vi "Get Substrings & Calculate CRC.vi"(8 "error in (no error)":errorcluster, 11 "Data In":string) -> (0 "error out":errorcluster, 2 "Analogs":string, 3 "Switches":string)   [LabVIEW 2015]
uses:
  <vilib>/Utility/error.llb/Error Cluster From Error Code.vi
  Inline CRC/CRC SubVIs/Wrappers/CRC-8-Maxim 1-Wire (DOW).vi
  <vilib>/ErrorRing/Error Ring.xnode
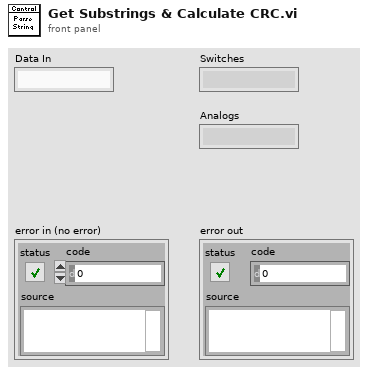
[diagram p1: front panel]
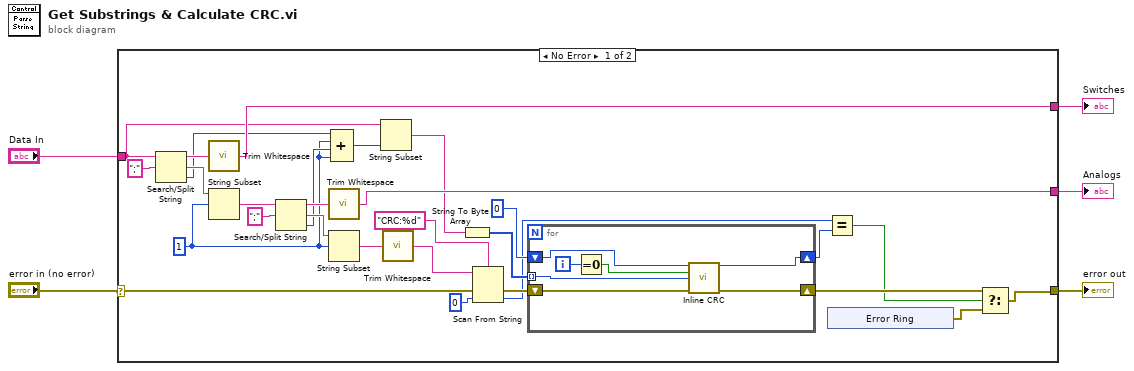
[diagram p0: block diagram]
diagram:
  n1 = case shown="No Error" "error in (no error)" {
    selector: "error in (no error)" -> [w10 w47]
    tunnel: [w32 _] -> w5
    tunnel: [w31 _] -> w4
    tunnel: "Data In" -> [w20 _]
    tunnel: [w8 w47] -> w2
    frame No Error {
      w21 = 1 ("offset (0)")
      n2 = Search/Split String(string=w20, search string/char (-)=";") -> (substring before match=w28:string, match + rest of string=w25:string, offset of match=w23:i32)  [unwired: 1 in]
      n3 = call <vilib>:"Trim Whitespace.vi"("string"=w28) -> ("trimmed string"=w31:string)  [unwired: 1 in]
      n4 = String Subset(string=w25, offset (0)=w21) -> (substring=w24:string)  [unwired: 1 in]
      n5 = Search/Split String(string=w24, search string/char (-)=";") -> (substring before match=w29:string, match + rest of string=w27:string, offset of match=w22:i32)  [unwired: 1 in]
      n6 = call <vilib>:"Trim Whitespace.vi"("string"=w29) -> ("trimmed string"=w32:string)  [unwired: 1 in]
      n7 = String Subset(string=w27, offset (0)=w21) -> (substring=w26:string)  [unwired: 1 in]
      n8 = Compound Arithmetic op=ADD(w23, w21, w22, w21) -> (w19:i32)
      n9 = String Subset(string=w20, length (rest)=w19) -> (substring=w18:string)  [unwired: 1 in]
      n10 = call <vilib>:"Trim Whitespace.vi"("string"=w26) -> ("trimmed string"=w15:string)  [unwired: 1 in]
      n11 = String To Byte Array(string=w18) -> (unsigned byte array=w17:u8[])
      n12 = Scan From String(format string="CRC:%d", input string=w15, error in=w10, default 1=u8 0 ("CRC")) -> (error out=w33:errorcluster, output 1=w13:u8)  [unwired: 1 in, 2 out]
      n13 = for {
        tunnel: w17 -> [w46] mode=indexing
        shift-right: [w44] -> w12
        shift-left: u8 0 ("CRC") -> [w45]
        shift-right: [w40] -> w9
        shift-left: w33 -> [w41]
        i -> [w43]
        n14 = Equal To 0?(x=w43) -> (x = 0?=w42:bool)
        n15 = call-poly "Inline CRC.vi"("CRC In"=w45, "Reset"=w42, "Data"=w46, "error in (no error)"=w41) -> ("CRC"=w44:u8, "error out"=w40:errorcluster)  [unwired: 10 in]
      }
      n16 = Equal?(x=w13, y=w12) -> (x = y?=w6:bool)
      n17 = xnode "Error Ring"() -> ("error out"=w7:errorcluster)
      n18 = Select(t=w9, s=w6, f=w7) -> (s? t:f=w8:errorcluster)
    }
    frame Error {
    }
  }
  "error out" <- w2
  "Analogs" <- w5
  "Switches" <- w4
